vi "Plot_em.vi"(0 "queue out":refnum<queue>, 1 "set bead as reference":bool, 2 "bead number":i32, 3 "delete bead & trace":bool, 4 "All beads":bool, 5 "Z only":bool, 7 "use reference":bool) -> (6 "Array":cluster{"time out":i32[], "xyz um out":dbl[]}[](array[cluster]), 8 "queue out 2":refnum<queue>)   [LabVIEW 2011]
uses:
  CP que.ctl
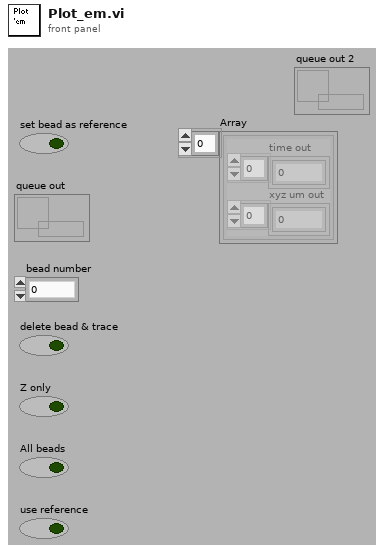
[diagram p1: front panel]
types:
  T1 = enum16{"init", "get", "set single frame", "set all"}
  T2 = typedef "IMAQ Image.ctl" = refnum<image>
  T3 = cluster{"front panel settings":cluster{"files":cluster{"LUT path":path, "Trace path":path, " folders #":i32, "base path":path, "use trace":bool, "use base":bool, "LUT tmp":i32, "Trace tmp":i32, "active path":path}, "Tracking":cluster{"RminZ (pix)":i32, "Rmax (pix)":i32, "angular pixel \ncoverage factor":dbl, "radial pixel \ncoverage factor":dbl}, "Frames":cluster{"Start frame":i32, "number of frames":u32, "display frame ":i32, "track every nd frame ":i32, "Track all frames":bool, "active frame":i32}, "Calibs":cluster{"Zlut number of steps":i32, "pix/um":dbl, "Z correction factor":dbl, "Zlut step size (um)":dbl, "ROI(pix)":i32}, "Beads":cluster{"number of ref beads":i32, "overlay":bool}, "Misc":cluster{"save images to new location":bool, "destination":path}}, "data":cluster{"Image":T2, "image size":i32[], "Bead Array":i32[][], "overlay image":T2, "# beads":i32, "Job list":string[][], "job running":bool, "job #":i32, "folders to go":i32}}
  T4 = typedef "CP que.ctl" = enum16{"idle", "settings", "display", "init", "set beads", "show LUT", "Zlut", "plot", "track", "do job", "joblist", "autoselect", "save", "stop"}
  T5 = cluster{"ROI1":i32, "Rmax (pix)":i32, "RminZ (pix)":i32, "LUTs":dbl[][][], "use trace":bool, "angular pixel\n coverage factor":dbl, "radial pixel\n coverage factor":dbl}
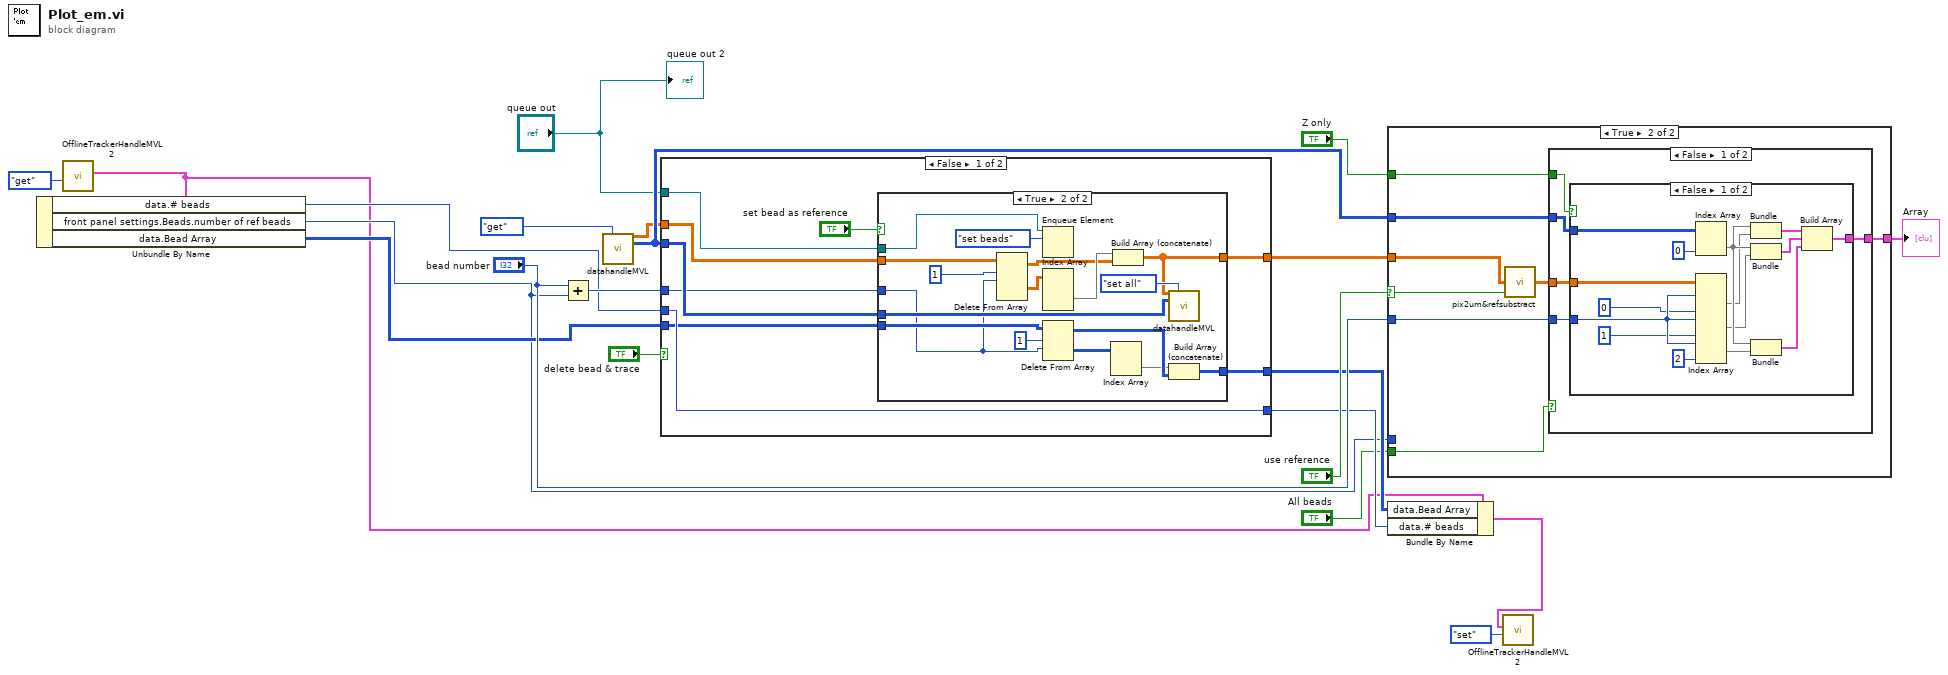
[diagram p0: block diagram]
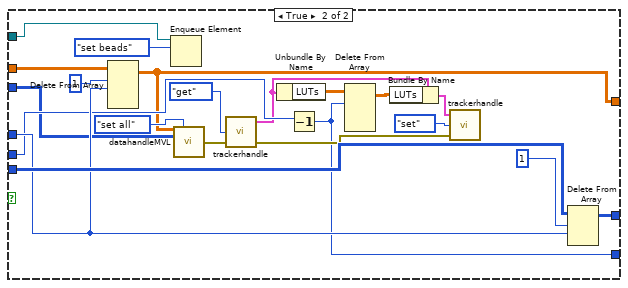
[diagram p3: hidden frame]
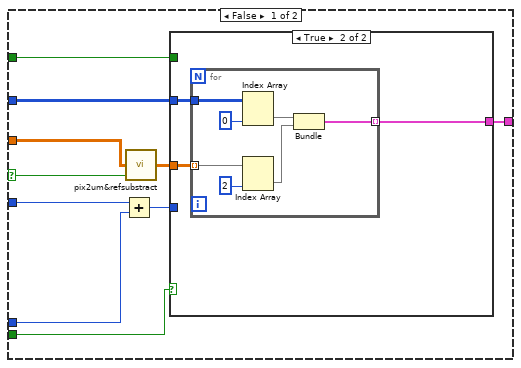
[diagram p4: hidden frame]
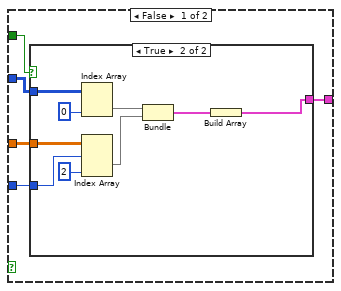
[diagram p5: hidden frame]
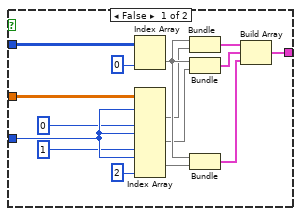
[diagram p6: hidden frame]
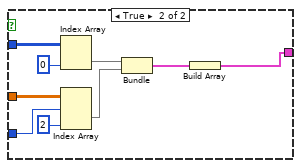
[diagram p7: hidden frame]
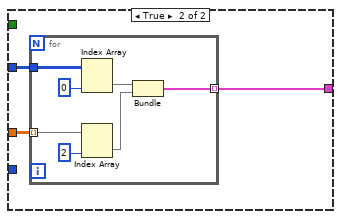
[diagram p8: hidden frame]
diagram:
  n1 = call "OfflineTrackerHandleMVL2.vi"("action"=enum16{"get", "set"}."get") -> ("out"=w1:T3)  [unwired: 5 in, 1 out]
  n2 = Unbundle By Name(w1) -> ("data.# beads"=w5:i32, "front panel settings.Beads.number of ref beads"=w4:i32, "data.Bead Array"=w6:i32[][])
  n3 = Add(x="bead number", y=w4) -> (x+y=w21:i32)
  n4 = call "datahandleMVL.vi"("action"=T1."get") -> ("XYZ out"=w13:dbl[][][], "time out"=w18:i32[][])  [unwired: 9 in, 4 out]
  n5 = case shown="False" "delete bead & trace" {
    tunnel: w13 -> [w28 w70]
    tunnel: [w27 w60] -> w14
    tunnel: w21 -> [w23 w67]
    tunnel: w6 -> [w25 w68]
    tunnel: [w24 w65] -> w15
    tunnel: w5 -> [w30 w64]
    tunnel: [w30 w50] -> w16
    tunnel: "queue out" -> [w22 w63]
    tunnel: w18 -> [w26 w59]
    frame False {
      n6 = case shown="True" "set bead as reference" {
        tunnel: w28 -> [w32 w47]
        tunnel: [w32 w43] -> w27
        tunnel: w26 -> [_ w42]
        tunnel: w25 -> [w31 w41]
        tunnel: [w31 w36] -> w24
        tunnel: w23 -> [_ w35]
        tunnel: w22 -> [_ w34]
        frame False {
        }
        frame True {
          n7 = Delete From Array(array=w47, length=1, index (dim 0)=w35) -> (deleted portion=w48:dbl[][][], array with subset deleted=w45:dbl[][][])  [unwired: 2 in]
          n8 = Enqueue Element(queue=w34, element=CP_que."set beads" ("CP que")) -> ()  [unwired: 1 in, 4 out]
          n9 = Index Array(array=w48) -> (element=w46:dbl[][])  [unwired: 3 in]
          n10 = Delete From Array(array=w41, length=1, index (row)=w35) -> (deleted portion=w38:i32[][], array with subset deleted=w39:i32[][])  [unwired: 1 in]
          n11 = Index Array(array=w38) -> (element=w37:i32[])  [unwired: 2 in]
          n12 = Build Array (concatenate)(w46, w45) -> (w43:dbl[][][])
          n13 = call "datahandleMVL.vi"("xyz array in"=w43, "action"=T1."set all", "Time array in"=w42) -> ()  [unwired: 7 in, 6 out]
          n14 = Build Array (concatenate)(w37, w39) -> (w36:i32[][])
        }
      }
    }
    frame True {
      n15 = Delete From Array(array=w70, length=1, index (dim 0)=w67) -> (array with subset deleted=w60:dbl[][][])  [unwired: 2 in, 1 out]
      n16 = Enqueue Element(queue=w63, element=CP_que."set beads" ("CP que")) -> ()  [unwired: 1 in, 4 out]
      n17 = call "datahandleMVL.vi"("xyz array in"=w60, "action"=T1."set all", "Time array in"=w59) -> ("error in 2"=w56:errorcluster)  [unwired: 7 in, 5 out]
      n18 = call "trackerhandle.vi"("error in"=w56, "action"=enum16{"get", "set"}."get") -> ("error out"=w58:errorcluster, "output Cluster"=w53:T5)  [unwired: 1 in, 1 out]
      n19 = Unbundle By Name(w53) -> ("LUTs"=w54:dbl[][][])
      n20 = Decrement(x=w64) -> (x-1=w50:i32)
      n21 = Delete From Array(array=w54, length=w50) -> (array with subset deleted=w51:dbl[][][])  [unwired: 3 in, 1 out]
      n22 = Bundle By Name(cluster=w53, "LUTs"=w51) -> (w52:T5)
      n23 = call "trackerhandle.vi"("error in"=w58, "action"=enum16{"get", "set"}."set", "input Cluster"=w52) -> ()  [unwired: 3 out]
      n24 = Delete From Array(array=w68, length=1, index (row)=w67) -> (array with subset deleted=w65:i32[][])  [unwired: 1 in, 1 out]
    }
  }
  n25 = case shown="True" "use reference" {
    selector: "use reference" -> [w76 w127]
    tunnel: [w80 w124] -> w8
    tunnel: "Z only" -> [w79 w126]
    tunnel: "All beads" -> [w78 w125]
    tunnel: "bead number" -> [w73 w120]
    tunnel: w14 -> [w75 w123]
    tunnel: w18 -> [w74 w122]
    tunnel: w4 -> [w71 _]
    frame False {
      n26 = Add(x=w73, y=w71) -> (x+y=w72:i32)
      n27 = call "pix2um&refsubstract.vi"("ref substract"=w76, "XYZ in"=w75) -> ("xyz um out"=w77:dbl[][][])  [unwired: 3 out]
      n28 = case shown="True" w78 {
        tunnel: w77 -> [w85 w112]
        tunnel: w74 -> [w84 w111]
        tunnel: [w82 w110] -> w80
        tunnel: w79 -> [w83 _]
        tunnel: w72 -> [w81 _]
        frame False {
          n29 = case shown="True" w83 {
            tunnel: w85 -> [w99 w107]
            tunnel: w81 -> [w97 w106]
            tunnel: w84 -> [w98 w105]
            tunnel: [w92 w103] -> w82
            frame False {
              n30 = Index Array(array=w98, index (col)=0 ("disabled index (col)")) -> (element=w96:i32[])  [unwired: 1 in]
              n31 = Index Array(array=w99, index (dim 0) #1=w97, index (dim 2) #1=0 ("disabled index (col)"), index (dim 0) #2=w97, index (dim 2) #2=1 ("disabled index (col)"), index (dim 0) #3=w97, index (dim 2) #3=2 ("disabled index (row)")) -> (element #1=w86:dbl[], element #2=w87:dbl[], element #3=w88:dbl[])  [unwired: 3 in]
              n32 = Bundle("time out"=w96, "xyz um out"=w86) -> (w95:cluster{"time out":i32[], "xyz um out":dbl[]})  [unwired: 1 out]
              n33 = Bundle("time out"=w96, "xyz um out"=w87) -> (w94:cluster{"time out":i32[], "xyz um out":dbl[]})  [unwired: 1 out]
              n34 = Bundle("time out"=w96, "xyz um out"=w88) -> (w93:cluster{"time out":i32[], "xyz um out":dbl[]})  [unwired: 1 out]
              n35 = Build Array(w95, w94, w93) -> (w92:cluster{"time out":i32[], "xyz um out":dbl[]}[])
            }
            frame True {
              n36 = Index Array(array=w105, index (col)=0 ("disabled index (col)")) -> (element=w108:i32[])  [unwired: 1 in]
              n37 = Index Array(array=w107, index (dim 0)=w106, index (dim 2)=2 ("disabled index (row)")) -> (element=w101:dbl[])  [unwired: 1 in]
              n38 = Bundle("time out"=w108, "xyz um out"=w101) -> (w104:cluster{"time out":i32[], "xyz um out":dbl[]})  [unwired: 1 out]
              n39 = Build Array(w104) -> (w103:cluster{"time out":i32[], "xyz um out":dbl[]}[])
            }
          }
        }
        frame True {
          n40 = for {
            tunnel: w112 -> [w119] mode=indexing
            tunnel: w111 -> [w118]
            tunnel: [w117] -> w110 mode=indexing
            n41 = Index Array(array=w118, index (col)=0 ("disabled index (col)")) -> (element=w116:i32[])  [unwired: 1 in]
            n42 = Index Array(array=w119, index (col)=2 ("disabled index (row)")) -> (element=w113:dbl[])  [unwired: 1 in]
            n43 = Bundle("time out"=w116, "xyz um out"=w113) -> (w117:cluster{"time out":i32[], "xyz um out":dbl[]})  [unwired: 1 out]
          }
        }
      }
    }
    frame True {
      n44 = call "pix2um&refsubstract.vi"("ref substract"=w127, "XYZ in"=w123) -> ("xyz um out"=w121:dbl[][][])  [unwired: 3 out]
      n45 = case shown="False" w125 {
        tunnel: w122 -> [w132 w159]
        tunnel: [w130 w158] -> w124
        tunnel: w126 -> [w131 _]
        tunnel: w121 -> [w129 w157]
        tunnel: w120 -> [w128 _]
        frame False {
          n46 = case shown="False" w131 {
            tunnel: w129 -> [w146 w154]
            tunnel: w128 -> [w144 w153]
            tunnel: w132 -> [w145 w152]
            tunnel: [w139 w150] -> w130
            frame False {
              n47 = Index Array(array=w145, index (col)=0 ("disabled index (col)")) -> (element=w143:i32[])  [unwired: 1 in]
              n48 = Index Array(array=w146, index (dim 0) #1=w144, index (dim 2) #1=0 ("disabled index (col)"), index (dim 0) #2=w144, index (dim 2) #2=1 ("disabled index (col)"), index (dim 0) #3=w144, index (dim 2) #3=2 ("disabled index (row)")) -> (element #1=w133:dbl[], element #2=w134:dbl[], element #3=w135:dbl[])  [unwired: 3 in]
              n49 = Bundle("time out"=w143, "xyz um out"=w133) -> (w142:cluster{"time out":i32[], "xyz um out":dbl[]})  [unwired: 1 out]
              n50 = Bundle("time out"=w143, "xyz um out"=w134) -> (w141:cluster{"time out":i32[], "xyz um out":dbl[]})  [unwired: 1 out]
              n51 = Bundle("time out"=w143, "xyz um out"=w135) -> (w140:cluster{"time out":i32[], "xyz um out":dbl[]})  [unwired: 1 out]
              n52 = Build Array(w142, w141, w140) -> (w139:cluster{"time out":i32[], "xyz um out":dbl[]}[])
            }
            frame True {
              n53 = Index Array(array=w152, index (col)=0 ("disabled index (col)")) -> (element=w155:i32[])  [unwired: 1 in]
              n54 = Index Array(array=w154, index (dim 0)=w153, index (dim 2)=2 ("disabled index (row)")) -> (element=w148:dbl[])  [unwired: 1 in]
              n55 = Bundle("time out"=w155, "xyz um out"=w148) -> (w151:cluster{"time out":i32[], "xyz um out":dbl[]})  [unwired: 1 out]
              n56 = Build Array(w151) -> (w150:cluster{"time out":i32[], "xyz um out":dbl[]}[])
            }
          }
        }
        frame True {
          n57 = for {
            tunnel: w157 -> [w166] mode=indexing
            tunnel: w159 -> [w165]
            tunnel: [w164] -> w158 mode=indexing
            n58 = Index Array(array=w165, index (col)=0 ("disabled index (col)")) -> (element=w163:i32[])  [unwired: 1 in]
            n59 = Index Array(array=w166, index (col)=2 ("disabled index (row)")) -> (element=w160:dbl[])  [unwired: 1 in]
            n60 = Bundle("time out"=w163, "xyz um out"=w160) -> (w164:cluster{"time out":i32[], "xyz um out":dbl[]})  [unwired: 1 out]
          }
        }
      }
    }
  }
  "Array" <- w8
  n61 = Bundle By Name(cluster=w1, "data.Bead Array"=w15, "data.# beads"=w16) -> (w2:T3)
  n62 = call "OfflineTrackerHandleMVL2.vi"("action"=enum16{"get", "set"}."set", "in"=w2) -> ()  [unwired: 4 in, 2 out]
  "queue out 2" <- "queue out"
